vi "ExSubNframeCol.vi"(2 "error in (no error)":errorcluster, 3 "Number of Images":u32=1 min=1 step=1, 4 "Handle Cluster":T1) -> (0 "error out":errorcluster, 1 "Handle Cluster":T1)   [LabVIEW 2010]
panel:
  # "ExSubNframeCol:\nThis is a sub VI that collects N frames from \nthe camera system. This assumes camera \nhas been setup and initialized and that the \nstart camera is done. It also assumes the \ncamera has circular buffer capabillities.\nThis is not true for all cameras, especially older \ncameras."
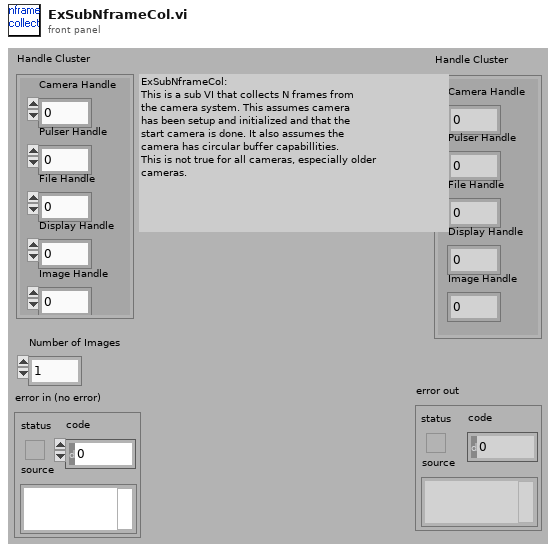
[diagram p1: front panel]
types:
  T1 = cluster{"Camera Handle":u32, "Pulser Handle":u32, "File Handle":u32, "Display Handle":u32, "Image Handle":u32}
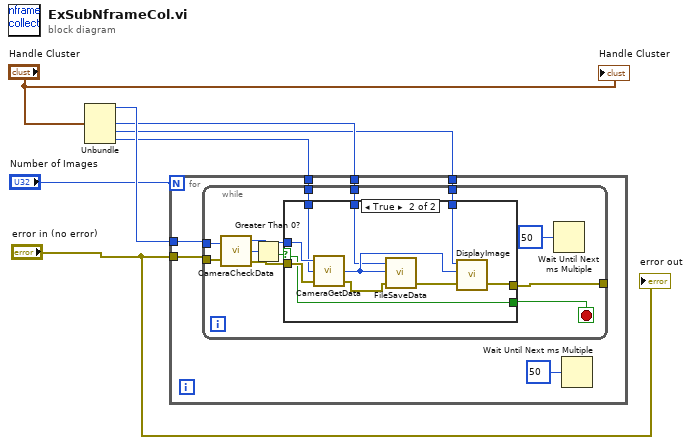
[diagram p0: block diagram]
diagram:
  n1 = Unbundle("Handle Cluster") -> ("Camera Handle"=w7:u32, "File Handle"=w6:u32, "Display Handle"=w5:u32, "Image Handle"=w4:u32)  [unwired: 1 out]
  n2 = for {
    N: "Number of Images" -> [_]
    tunnel: w7 -> [w13]
    tunnel: w6 -> [w12]
    tunnel: w5 -> [w11]
    tunnel: w4 -> [w10]
    tunnel: "error in (no error)" -> [w9]
    n3 = while {
      tunnel: w9 -> [w24]
      tunnel: w13 -> [w23]
      tunnel: [w18] -> _
      tunnel: w12 -> [w17]
      tunnel: w11 -> [w16]
      tunnel: w10 -> [w15]
      stop <- w19 stop-if-true
      n4 = call <userlib>:"CameraCheckData.vi"("Camera Handle"=w23, "error in"=w24) -> ("Camera Handle"=w21:u32, "Number Of Frames Available"=w25:i32, "error out"=w20:errorcluster)
      n5 = Greater Than 0?(x=w25) -> (x > 0?=w22:bool)
      n6 = case shown="True" w22 {
        selector: w22 -> [w26 w35]
        tunnel: w21 -> [_ w37]
        tunnel: w20 -> [w27 w36]
        tunnel: [w26 w35] -> w19
        tunnel: [w27 w32] -> w18
        tunnel: w17 -> [_ w30]
        tunnel: w16 -> [_ w29]
        tunnel: w15 -> [_ w28]
        frame False {
        }
        frame True {
          n7 = call <userlib>:"CameraGetData.vi"("error in"=w36, "Data Handle"=w28, "Camera Handle"=w37) -> ("error out"=w34:errorcluster, "Data Handle"=w31:u32)  [unwired: 1 out]
          n8 = call <userlib>:"FileSaveData.vi"("error in"=w34, "Image Handle"=w31, "File Handle"=w30) -> ("error out"=w33:errorcluster)  [unwired: 1 out]
          n9 = call <userlib>:"DisplayImage.vi"("error in"=w33, "Image Handle"=w31, "Display Handle"=w29) -> ("error out"=w32:errorcluster)  [unwired: 1 in, 1 out]
        }
      }
      n10 = Wait Until Next ms Multiple(millisecond multiple=u32 50) -> ()  [unwired: 1 out]
    }
    n11 = Wait Until Next ms Multiple(millisecond multiple=u32 50) -> ()  [unwired: 1 out]
  }
  "error out" <- "error in (no error)"
  "Handle Cluster" <- "Handle Cluster"
